vi "Translator.MainGui.vi"(6 "~Do not save font? (F)":bool, 7 "~init (F)":bool, 8 "~error in":errorcluster, 10 "~Language in use":string="English", 11 "~Translation folder":path=path "D:/PL_0125_Sapphire_Automation_branches/SOFTWARE_v1.1-Translation/settings") -> (0 "~error out":errorcluster, 1 "~restart?":bool, 2 "~font name":string, 4 "~flag small":picture)   [LabVIEW 2016]
uses:
  <vilib>/Utility/miscctls.llb/LVBoundsTypeDef.ctl
  Config/Config.Global.vi
  Translator.Global.vi
panel:
  out "~progressbar2":i32(slide) scale=-1.1..6.0
  out "~progressbar1":i32(slide) scale=-1.1..-1.0
  out "Message":string
  out "~flag":picture
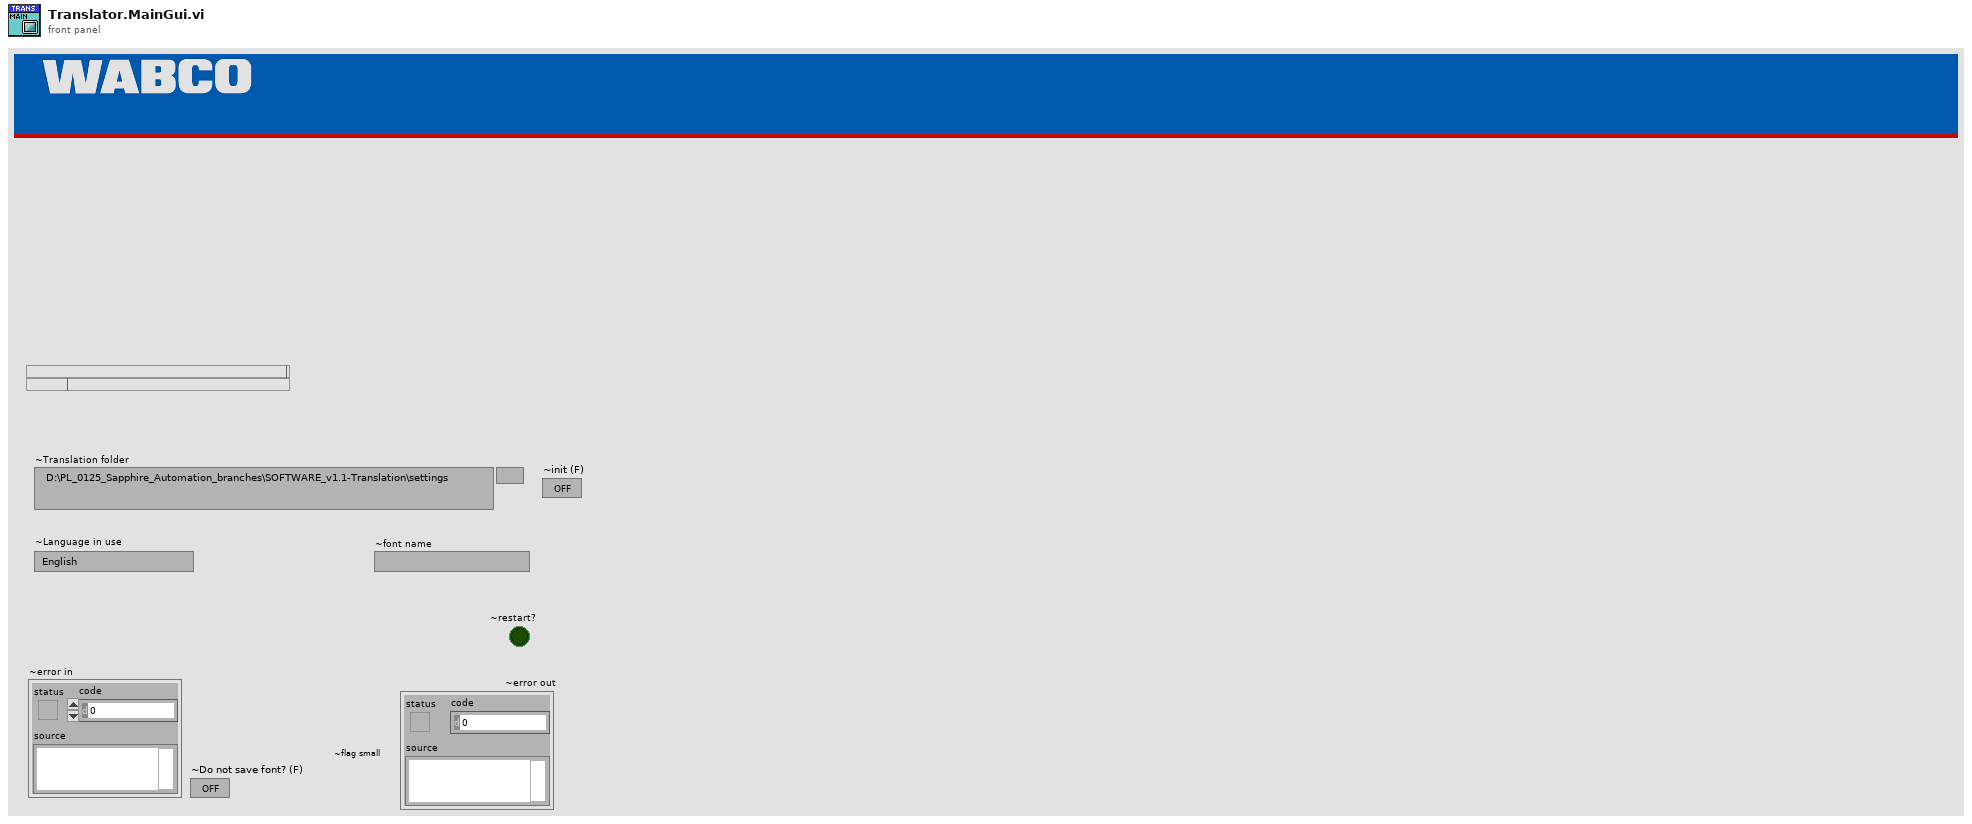
[diagram p1: front panel]
types:
  T1 = typedef "LVBoundsTypeDef.ctl" = cluster{"Width":u32, "Height":u32}
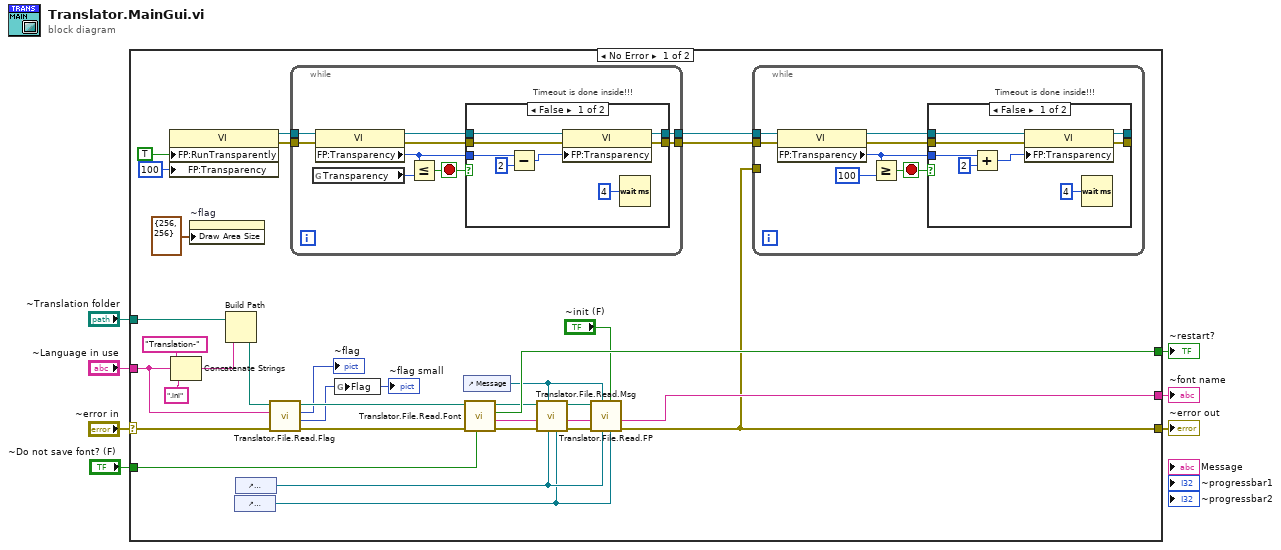
[diagram p0: block diagram]
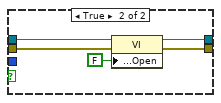
[diagram p2: hidden frame]
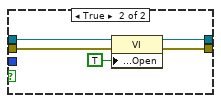
[diagram p3: hidden frame]
diagram:
  n1 = case shown="No Error" "~error in" {
    selector: "~error in" -> [w27 w77]
    tunnel: "~Translation folder" -> [w23 _]
    tunnel: [w15 w77] -> w4
    tunnel: "~Language in use" -> [w26 _]
    tunnel: [w18 _] -> w3
    tunnel: [w29 _] -> w2
    tunnel: "~Do not save font? (F)" -> [w24 _]
    frame No Error {
      n2 = property class="VI"("FP:RunTransparently"=TRUE ("Front Panel Window:Run VI Transparently"), "FP:Transparency"=u8 100 ("Front Panel Window:Transparency")) -> (reference out=w20:refnum<vi>, error out=w21:errorcluster)  [unwired: 2 in]
      n3 = Concatenate Strings("Translation-" ("string"), w26, ".ini" ("string")) -> (w32:string)
      n4 = property on="~flag" class="Pict"("Draw Area Size"=T1 {"Width"=256, "Height"=256}) -> ()  [unwired: 2 in, 2 out]
      n5 = Build Path(base path=w23, name or relative path=w32) -> (appended path=w28:path)
      n6 = control-ref of="~progressbar2"() -> (w30:refnum<vi>)
      n7 = control-ref of="~progressbar1"() -> (w31:refnum<vi>)
      n8 = call "Translator.File.Read.Flag.vi"("error in"=w27, "Language in use"=w26, "Translation file"=w28) -> ("error out"=w10:errorcluster, "~flag small"=w8:picture, "~flag"=→"~flag":picture)  [unwired: 6 in]
      "~flag small" <- w8
      n9 = while {
        tunnel: w21 -> [w58]
        tunnel: w20 -> [w57]
        tunnel: [w56] -> w17
        tunnel: [w55] -> w16
        stop <- w59 stop-if-true
        # "Timeout is done inside!!!"
        n10 = global read "Config.Global.vi" "Transparency"() -> (w63:u8)
        n11 = property class="VI"(reference=w57, error in=w58) -> (reference out=w61:refnum<vi>, error out=w62:errorcluster, "FP:Transparency"=w60:u8)
        n12 = Less Or Equal?(x=w60, y=w63) -> (x <= y?=w59:bool)
        n13 = case shown="False" w59 {
          tunnel: w62 -> [w71 w76]
          tunnel: w61 -> [w70 w75]
          tunnel: w60 -> [w69 _]
          tunnel: [w67 w74] -> w55
          tunnel: [w66 w73] -> w56
          frame False {
            n14 = Subtract(x=w69, y=u8 2 ("x")) -> (x-y=w68:u8)
            n15 = property class="VI"(reference=w70, error in=w71, "FP:Transparency"=w68) -> (reference out=w66:refnum<vi>, error out=w67:errorcluster)
            n16 = Wait (ms)(milliseconds to wait=u32 4) -> ()  [unwired: 1 out]
          }
          frame True {
            n17 = property class="VI"(reference=w75, error in=w76, "Front Panel.Open"=TRUE ("Front Panel Window:Open")) -> (reference out=w73:refnum<vi>, error out=w74:errorcluster)
          }
        }
      }
      n18 = global write "Translator.Global.vi" "Flag"(w8) -> ()
      n19 = control-ref of="Message"() -> (w14:refnum<vi>)
      n20 = call "Translator.File.Read.Font.vi"("Do not save font? (F)"=w24, "error in"=w10, "Translation file"=w28) -> ("error out"=w13:errorcluster, "font name"=w18:string, "restart required?"=w29:bool)  [unwired: 6 in]
      n21 = call "Translator.File.Read.Msg.vi"("progressbar2"=w30, "progressbar1"=w31, "Message"=w14, "error in"=w13, "Translation folder"=w28) -> ("error out"=w12:errorcluster)  [unwired: 6 in]
      n22 = call "Translator.File.Read.FP.vi"("progressbar2"=w30, "init"="~init (F)", "progressbar1"=w31, "Message"=w14, "error in"=w12, "font name"=w18, "Translation file"=w28) -> ("error out"=w15:errorcluster)  [unwired: 4 in]
      n23 = while {
        tunnel: w16 -> [w37]
        tunnel: w17 -> [w36]
        tunnel: w15 -> [_]
        stop <- w38 stop-if-true
        # "Timeout is done inside!!!"
        n24 = property class="VI"(reference=w36, error in=w37) -> (reference out=w40:refnum<vi>, error out=w41:errorcluster, "FP:Transparency"=w39:u8)
        n25 = Greater Or Equal?(x=w39, y=u8 100) -> (x >= y?=w38:bool)
        n26 = case shown="False" w38 {
          tunnel: w41 -> [w49 w54]
          tunnel: w40 -> [w48 w53]
          tunnel: w39 -> [w47 _]
          tunnel: [w46 w52] -> _
          tunnel: [w45 w51] -> _
          frame False {
            n27 = Add(x=w47, y=u8 2 ("x")) -> (x+y=w42:u8)
            n28 = property class="VI"(reference=w48, error in=w49, "FP:Transparency"=w42) -> (reference out=w45:refnum<vi>, error out=w46:errorcluster)
            n29 = Wait (ms)(milliseconds to wait=u32 4) -> ()  [unwired: 1 out]
          }
          frame True {
            n30 = property class="VI"(reference=w53, error in=w54, "Front Panel.Open"=FALSE ("Front Panel Window:Open")) -> (reference out=w51:refnum<vi>, error out=w52:errorcluster)
          }
        }
      }
    }
    frame Error {
    }
  }
  "~error out" <- w4
  "~font name" <- w3
  "~restart?" <- w2
